vi "Begin.vi"(8 "error in":errorcluster) -> (0 "error out":errorcluster)   [LabVIEW 2020]
doc: "Called before other user functions, this VI is expected to open initial I/O refnums, load in file data, and do all program initialization. Notice that the <B>error out</B> terminal is simply used for data flow. Wiring it to other structures or subVIs ensures that this VI runs first."
uses:
  <vilib>/Rock Robotics/WPI/DriverStation/WPI_DriverStationRobotMode2.ctl
  <vilib>/Rock Robotics/WPI/Joystick/WPI_JoystickDeviceEnum.ctl
  <vilib>/Rock Robotics/WPI/ThirdParty/REV Robotics/REVLib/Typedef/Spark MAX Control Type.ctl
  <vilib>/Rock Robotics/WPI/ThirdParty/Sensors/navX/_TypeDefs/FRIC_navX_DeviceNumbersTypeDef.ctl
  Robot Global Data.vi
  <vilib>/Rock Robotics/Network Tables/NT Write String Array.vi
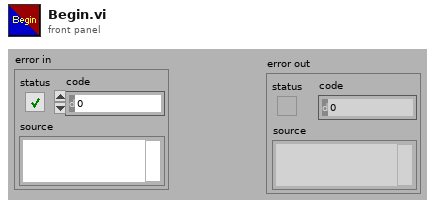
[diagram p1: front panel]
types:
  T1 = typedef "FRIC_navX_DeviceNumbersTypeDef.ctl" = enum16{"Dev0", "Dev1", "Dev2", "Dev3"}
  T2 = typedef "Spark MAX Control Type.ctl" = enum16{"Percent VBus", "Voltage", "Velocity", "Position", "Smart Motion", "Current", "Smart Velocity"}
  T3 = typedef "WPI_JoystickDeviceEnum.ctl" = enum16{"USB 0", "USB 1", "USB 2", "USB 3", "USB 4", "USB 5"}
  T4 = typedef "WPI_DriverStationRobotMode2.ctl" = enum16{"Autonomous Disabled", "Autonomous Enabled", "Teleop Disabled", "Teleop Enabled", "Disconnected", "Finish", "Test Disabled", "Test Enabled", "Emergency Stopped"}
  T5 = typedef "WPI_JoystickDevRef.ctl" = cluster{"Device":T3}
  T6 = typedef "WPI_MotorControlDeviceRef.ctl" = cluster{"DeviceStatus":errorcluster, "Type":T7, "PWM":cluster{"PWM Channel":T8, "DeadBand":T9}, "CAN":cluster{"Device Number":u8, "SetOutput VI Ref":variant, "GetOutput VI Ref":variant, "Enable VI Ref":variant, "Disable VI Ref":variant, "Data":variant}, "Invert":bool, "DIO PWM":cluster{"PWM \"Enable\" Channel":T8, "DIOChannel":T10, "PWM Rate":dbl}}
  T7 = typedef "WPI_MotorControlType.ctl" = enum16{"PWM", "CAN", "DIO PWM"}
  T8 = typedef "FPGA_DIOPWMChannel.ctl" = enum8{"PWM 0", "PWM 1", "PWM 2", "PWM 3", "PWM 4", "PWM 5", "PWM 6", "PWM 7", "PWM 8", "PWM 9", "PWM MXP 0", "PWM MXP 1", "PWM MXP 2", "PWM MXP 3", "PWM MXP 4", "PWM MXP 5", "PWM MXP 6", "PWM MXP 7", "PWM MXP 8", "PWM MXP 9", "Invalid"}
  T9 = typedef "WPI_PWMDeadband.ctl" = cluster{"Name":string, "maxPositivePwm":i32, "minPositivePwm":i32, "centerPwm":i32, "maxNegativePwm":i32, "minNegativePwm":i32, "angularRange":u16}
  T10 = typedef "FPGA_DIOChannel.ctl" = enum8{"DIO 0", "DIO 1", "DIO 2", "DIO 3", "DIO 4", "DIO 5", "DIO 6", "DIO 7", "DIO 8", "DIO 9", "DIO MXP 0", "DIO MXP 1", "DIO MXP 2", "DIO MXP 3", "DIO MXP 4", "DIO MXP 5", "DIO MXP 6", "DIO MXP 7", "DIO MXP 8", "DIO MXP 9", "DIO MXP 10", "DIO MXP 11", "DIO MXP 12", "DIO MXP 13", "DIO MXP 14", "DIO MXP 15", "SPI Port CS1", "SPI Port CS2", "SPI Port CS3", "SPI Port MISO", "SPI Port MOSI", "Invalid"}
  T11 = typedef "CTRE_Phoenix_CANcoder_DeviceRef.ctl" = cluster{"DeviceStatus":errorcluster, "Device Number":u8, "Handle":u64, "UsageFrame":u32, "Library Path":path}
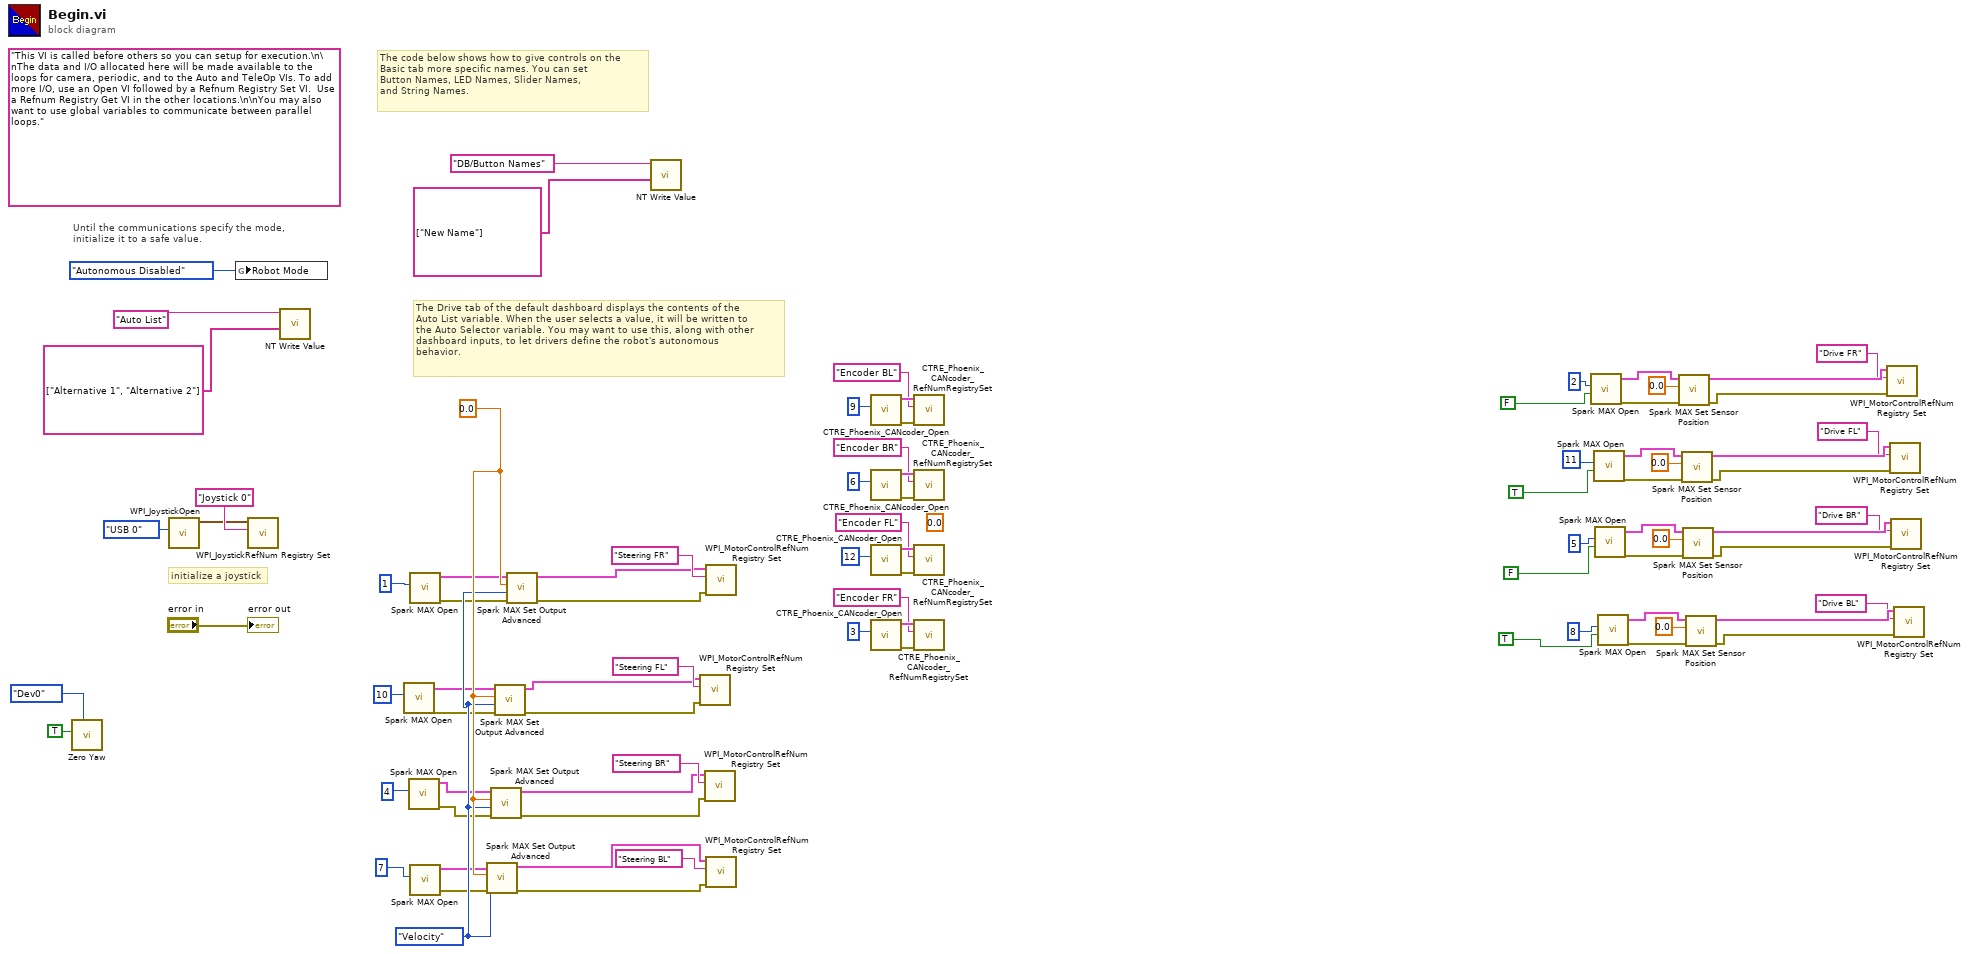
[diagram p0: block diagram]
diagram:
  w23 = Spark_MAX_Control_Type."Velocity" ("Control Mode")
  (unwired) 0.0 ("Position")
  w24 = 0.0 ("New Position")
  (unwired) "This VI is called before others so you can setup for execution.\n\nThe data and I/O allocated here will be made available to the loops for camera, periodic, and to the Auto and TeleOp VIs. To add more I/O, use an Open VI followed by a Refnum Registry Set VI.  Use a Refnum Registry Get VI in the other locations.\n\nYou may also want to use global variables to communicate between parallel loops."
  # "The Drive tab of the default dashboard displays the contents of the\nAuto List variable. When the user selects a value, it will be written to\nthe Auto Selector variable. You may want to use this, along with other\ndashboard inputs, to let drivers define the robot's autonomous\nbehavior."
  # "The code below shows how to give controls on the\nBasic tab more specific names. You can set\nButton Names, LED Names, Slider Names,\nand String Names."
  # "initialize a joystick"
  # "Until the communications specify the mode,\ninitialize it to a safe value."
  n1 = call <vilib>:"Zero Yaw.vi"("Device Number"=FRIC_navX_DeviceNumbersTypeDef."Dev0", "Zero"=TRUE) -> ()  [unwired: 10 in]
  n2 = call <vilib>:"WPI_JoystickOpen.vi"("JoystickDevice"=WPI_JoystickDeviceEnum."USB 0") -> ("JoystickDevRef"=w83:T5)  [unwired: 10 in]
  n3 = global write "Robot Global Data.vi" "Robot Mode"(WPI_DriverStationRobotMode2."Autonomous Disabled" ("Robot Mode")) -> ()
  n4 = call <vilib>:"WPI_JoystickRefNum Registry Set.vi"("refnum name"="Joystick 0", "JoystickDevRef"=w83) -> ()  [unwired: 8 in, 2 out]
  n5 = call-poly <vilib>:"NT Write Value.vi"("value"=string[] ["Alternative 1", "Alternative 2"] ("String Array"), "name"="Auto List" ("Name")) -> ()  [unwired: 9 in, 1 out]
  n6 = call <vilib>:"Spark MAX Open.vi"("Device Number"=u8 10) -> ("error out"=w19:errorcluster, "MotorControlDeviceRef"=w20:T6)  [unwired: 9 in]
  n7 = call <vilib>:"Spark MAX Open.vi"("Device Number"=u8 4) -> ("error out"=w17:errorcluster, "MotorControlDeviceRef"=w18:T6)  [unwired: 9 in]
  n8 = call <vilib>:"Spark MAX Open.vi"("Device Number"=u8 1) -> ("error out"=w21:errorcluster, "MotorControlDeviceRef"=w22:T6)  [unwired: 9 in]
  n9 = call <vilib>:"Spark MAX Open.vi"("Device Number"=u8 7) -> ("error out"=w15:errorcluster, "MotorControlDeviceRef"=w16:T6)  [unwired: 9 in]
  n10 = call <vilib>:"Spark MAX Set Output Advanced.vi"("error in (no error)"=w15, "Control Mode"=w23, "Setpoint"=w24, "MotorControlDevRef"=w16) -> ("error out"=w13:errorcluster, "MotorControlDevRef"=w14:T6)  [unwired: 6 in]
  n11 = call <vilib>:"Spark MAX Set Output Advanced.vi"("error in (no error)"=w17, "Control Mode"=w23, "Setpoint"=w24, "MotorControlDevRef"=w18) -> ("error out"=w11:errorcluster, "MotorControlDevRef"=w12:T6)  [unwired: 6 in]
  n12 = call <vilib>:"Spark MAX Set Output Advanced.vi"("error in (no error)"=w19, "Control Mode"=w23, "Setpoint"=w24, "MotorControlDevRef"=w20) -> ("error out"=w9:errorcluster, "MotorControlDevRef"=w10:T6)  [unwired: 6 in]
  n13 = call <vilib>:"Spark MAX Set Output Advanced.vi"("error in (no error)"=w21, "Control Mode"=w23, "Setpoint"=w24, "MotorControlDevRef"=w22) -> ("error out"=w7:errorcluster, "MotorControlDevRef"=w8:T6)  [unwired: 6 in]
  n14 = call-poly <vilib>:"NT Write Value.vi"("value"=string[] ["New Name"], "name"="DB/Button Names" ("Name")) -> ()  [unwired: 9 in, 1 out]
  n15 = call <vilib>:"WPI_MotorControlRefNum Registry Set.vi"("error in (no error)"=w9, "refnum name"="Steering FL", "MotorControlDevRef"=w10) -> ()  [unwired: 7 in, 2 out]
  n16 = call <vilib>:"WPI_MotorControlRefNum Registry Set.vi"("error in (no error)"=w11, "refnum name"="Steering BR", "MotorControlDevRef"=w12) -> ()  [unwired: 7 in, 2 out]
  n17 = call <vilib>:"WPI_MotorControlRefNum Registry Set.vi"("error in (no error)"=w7, "refnum name"="Steering FR", "MotorControlDevRef"=w8) -> ()  [unwired: 7 in, 2 out]
  n18 = call <vilib>:"WPI_MotorControlRefNum Registry Set.vi"("error in (no error)"=w13, "refnum name"="Steering BL", "MotorControlDevRef"=w14) -> ()  [unwired: 7 in, 2 out]
  n19 = call <vilib>:"CTRE_Phoenix_CANcoder_Open.vi"("Device Number"=u8 9) -> ("error out"=w64:errorcluster, "CTRE_CANcoder_DeviceRef"=w63:T11)  [unwired: 9 in]
  n20 = call <vilib>:"CTRE_Phoenix_CANcoder_Open.vi"("Device Number"=u8 6) -> ("error out"=w68:errorcluster, "CTRE_CANcoder_DeviceRef"=w67:T11)  [unwired: 9 in]
  n21 = call <vilib>:"CTRE_Phoenix_CANcoder_Open.vi"("Device Number"=u8 12) -> ("error out"=w72:errorcluster, "CTRE_CANcoder_DeviceRef"=w71:T11)  [unwired: 9 in]
  n22 = call <vilib>:"CTRE_Phoenix_CANcoder_Open.vi"("Device Number"=u8 3) -> ("error out"=w76:errorcluster, "CTRE_CANcoder_DeviceRef"=w75:T11)  [unwired: 9 in]
  n23 = call <vilib>:"CTRE_Phoenix_CANcoder_RefNumRegistrySet.vi"("error in (no error)"=w64, "refnum name"="Encoder BL", "CTRE_CANcoder_DeviceRef"=w63) -> ()  [unwired: 7 in, 2 out]
  n24 = call <vilib>:"CTRE_Phoenix_CANcoder_RefNumRegistrySet.vi"("error in (no error)"=w68, "refnum name"="Encoder BR", "CTRE_CANcoder_DeviceRef"=w67) -> ()  [unwired: 7 in, 2 out]
  n25 = call <vilib>:"CTRE_Phoenix_CANcoder_RefNumRegistrySet.vi"("error in (no error)"=w72, "refnum name"="Encoder FL", "CTRE_CANcoder_DeviceRef"=w71) -> ()  [unwired: 7 in, 2 out]
  n26 = call <vilib>:"CTRE_Phoenix_CANcoder_RefNumRegistrySet.vi"("error in (no error)"=w76, "refnum name"="Encoder FR", "CTRE_CANcoder_DeviceRef"=w75) -> ()  [unwired: 7 in, 2 out]
  n27 = call <vilib>:"Spark MAX Open.vi"("Invert"=FALSE, "Device Number"=u8 2) -> ("error out"=w50:errorcluster, "MotorControlDeviceRef"=w51:T6)  [unwired: 8 in]
  n28 = call <vilib>:"Spark MAX Open.vi"("Invert"=TRUE, "Device Number"=u8 11) -> ("error out"=w45:errorcluster, "MotorControlDeviceRef"=w46:T6)  [unwired: 8 in]
  n29 = call <vilib>:"Spark MAX Open.vi"("Invert"=FALSE, "Device Number"=u8 5) -> ("error out"=w40:errorcluster, "MotorControlDeviceRef"=w41:T6)  [unwired: 8 in]
  n30 = call <vilib>:"Spark MAX Open.vi"("Invert"=TRUE, "Device Number"=u8 8) -> ("error out"=w35:errorcluster, "MotorControlDeviceRef"=w36:T6)  [unwired: 8 in]
  n31 = call <vilib>:"Spark MAX Set Sensor Position.vi"("error in"=w50, "Position"=0.0 ("New Position"), "MotorControlDeviceRef"=w51) -> ("error out"=w49:errorcluster, "MotorControlDeviceRef"=w48:T6)  [unwired: 7 in]
  n32 = call <vilib>:"Spark MAX Set Sensor Position.vi"("error in"=w45, "Position"=0.0 ("New Position"), "MotorControlDeviceRef"=w46) -> ("error out"=w44:errorcluster, "MotorControlDeviceRef"=w43:T6)  [unwired: 7 in]
  n33 = call <vilib>:"Spark MAX Set Sensor Position.vi"("error in"=w40, "Position"=0.0 ("New Position"), "MotorControlDeviceRef"=w41) -> ("error out"=w39:errorcluster, "MotorControlDeviceRef"=w38:T6)  [unwired: 7 in]
  n34 = call <vilib>:"Spark MAX Set Sensor Position.vi"("error in"=w35, "Position"=0.0 ("New Position"), "MotorControlDeviceRef"=w36) -> ("error out"=w34:errorcluster, "MotorControlDeviceRef"=w33:T6)  [unwired: 7 in]
  n35 = call <vilib>:"WPI_MotorControlRefNum Registry Set.vi"("error in (no error)"=w49, "refnum name"="Drive FR", "MotorControlDevRef"=w48) -> ()  [unwired: 7 in, 2 out]
  n36 = call <vilib>:"WPI_MotorControlRefNum Registry Set.vi"("error in (no error)"=w44, "refnum name"="Drive FL", "MotorControlDevRef"=w43) -> ()  [unwired: 7 in, 2 out]
  n37 = call <vilib>:"WPI_MotorControlRefNum Registry Set.vi"("error in (no error)"=w39, "refnum name"="Drive BR", "MotorControlDevRef"=w38) -> ()  [unwired: 7 in, 2 out]
  n38 = call <vilib>:"WPI_MotorControlRefNum Registry Set.vi"("error in (no error)"=w34, "refnum name"="Drive BL", "MotorControlDevRef"=w33) -> ()  [unwired: 7 in, 2 out]
  "error out" <- "error in"
